vi "Handling Mouse Wheel Events.vi"() -> ()   [LabVIEW 2023]
doc: "Demonstrates the Mouse Wheel user interface event."
panel:
  in  "Stop":bool
  in  "Picture":picture
  # "Overview: Demonstrates the use of the Mouse Wheel event.\nRequirements: Mouse with wheel\nInstructions:\n1. Run the VI.\n2. Place the mouse cursor over the picture.\n3. Operate the mouse wheel to zoom in and out on the picture.\n4. Click Stop to stop the VI."
  # "Notes:\n\nThe image in this Picture is the default value of the control.\n\nThis VI has its panel's scrollbars hidden so that the wheel does not scroll the panel. Select File > VI Properties > Window Appearance and click the Customize button to configure the scrollbar visibility on the VI.\n\nThe Picture has its built-in mouse wheel behavior set to None. Since the picture control does not have its scrollbars visible, this is not functionally necessary, but is a good practice. Right-click on the Picture and select Properties > Key Navigation to configure the built-in mouse wheel behavior. Note that the Key Navigation page is disabled for indicators."
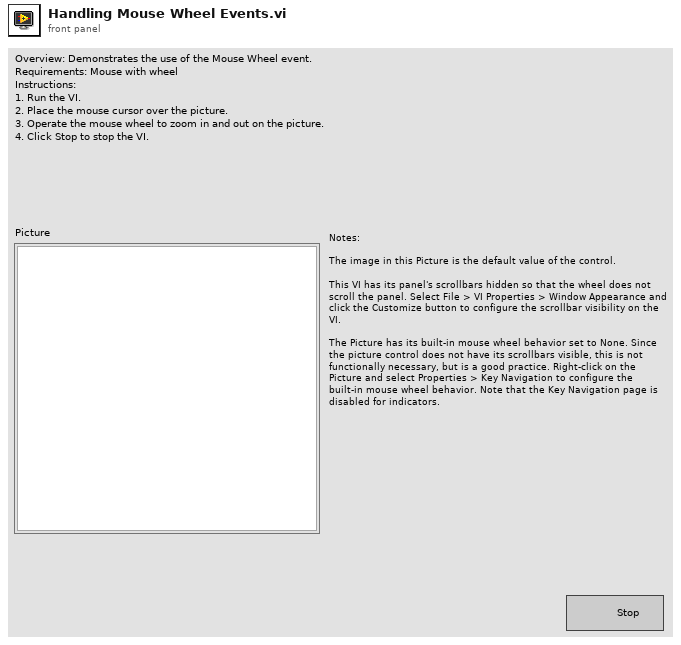
[diagram p1: front panel]
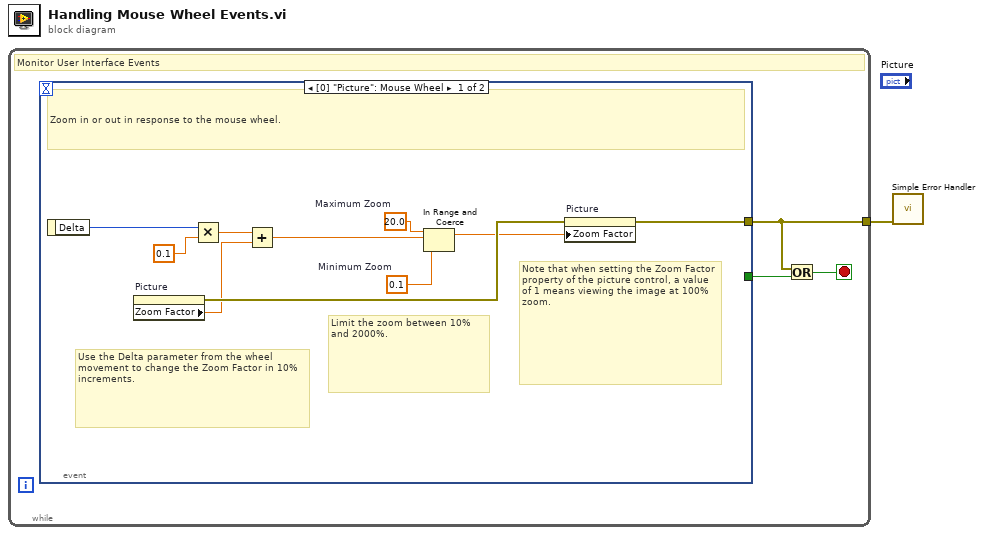
[diagram p0: block diagram]
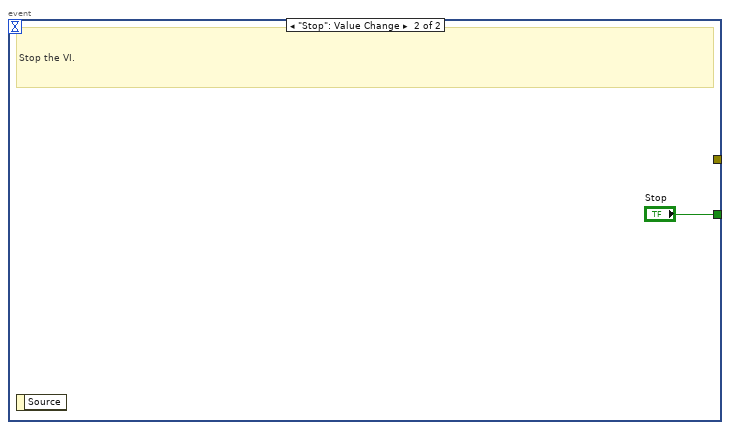
[diagram p2: hidden frame]
diagram:
  n1 = while {
    tunnel: [w2] -> w1
    stop <- w3 stop-if-true
    # "Monitor User Interface Events"
    n2 = event shown="[0] \"Picture\": Mouse Wheel" {
      selector: _ -> [_ _]
      dyn-events: _ -> [_ _]
      timeout: _ -> [_ _]
      tunnel: [_ "Stop"] -> w4
      tunnel: [w13 _] -> w2
      event "Picture": Mouse Wheel {
        w7 = 0.1  # Minimum Zoom
        w8 = 20.0  # Maximum Zoom
        # "Note that when setting the Zoom Factor property of the picture control, a value of 1 means viewing the image at 100% zoom."
        # "Use the Delta parameter from the wheel movement to change the Zoom Factor in 10% increments."
        # "Limit the zoom between 10% and 2000%."
        # "Zoom in or out in response to the mouse wheel."
        n3 = event-data() -> ("Delta"=w12:i32)  [unwired: 1 in]
        n4 = property on="Picture" class="Picture"() -> (error out=w14:errorcluster, "Zoom Factor"=w6:sgl)  [unwired: 2 in, 1 out]
        n5 = Multiply(x=w12, y=0.1) -> (x*y=w10:dbl)
        n6 = Add(x=w10, y=w6) -> (x+y=w9:dbl)
        n7 = In Range and Coerce(upper limit=w8, x=w9, lower limit=w7) -> (coerced(x)=w5:dbl)  [unwired: 1 out]
        n8 = property on="Picture" class="Picture"(error in=w14, "Zoom Factor"=w5) -> (error out=w13:errorcluster)  [unwired: 1 in, 1 out]
      }
      event "Stop": Value Change {
        # "Stop the VI."
        n9 = event-data() -> ()  [unwired: 1 in, 1 out]
      }
    }
    n10 = Or(x=w2, y=w4) -> (x .or. y?=w3:bool)
  }
  n11 = call <vilib>:"Simple Error Handler.vi"("error in (no error)"=w1) -> ()  [unwired: 4 in, 5 out]
